vi "encodeArrayBoolean.vi"(8 "error in (no error)":errorcluster, 11 "Boolean Array":bool[](array[boolean])) -> (0 "error out":errorcluster, 3 "MessagePack":u8[](array[numeric]) format="%.0x")   [LabVIEW 2015, in "MsgPack.lvlib"]
uses:
  MsgPack.lvlib
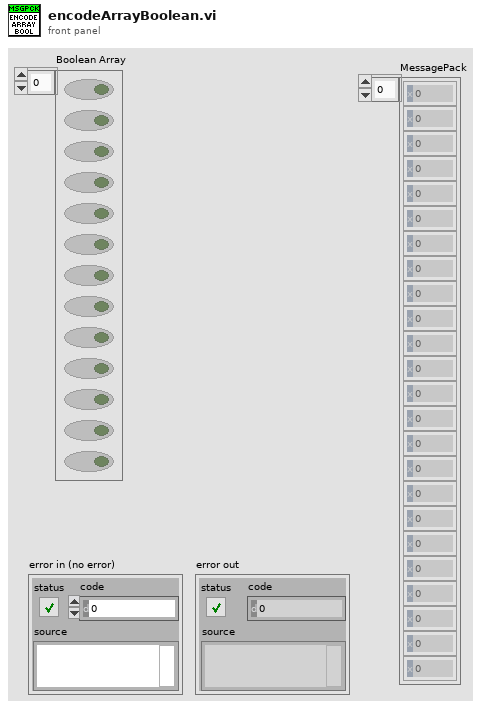
[diagram p1: front panel]
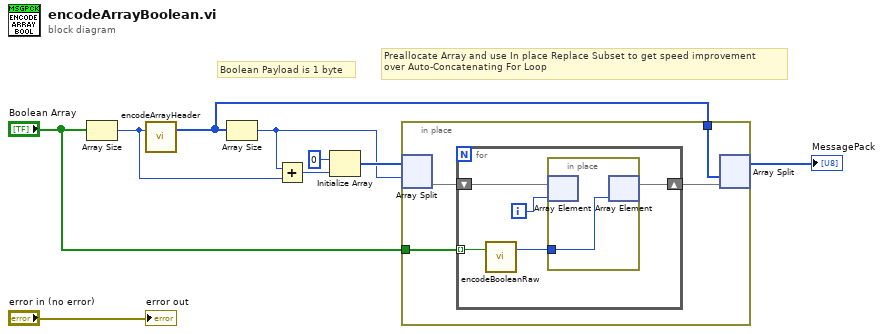
[diagram p0: block diagram]
diagram:
  # "Preallocate Array and use In place Replace Subset to get speed improvement\nover Auto-Concatenating For Loop"
  # "Boolean Payload is 1 byte"
  n1 = Array Size(array="Boolean Array") -> (size(s)=w2:i32)
  n2 = call "encodeArrayHeader.vi"("Number of Elements"=w2) -> ("array header"=w5:u8[])  [unwired: 2 in]
  n3 = Array Size(array=w5) -> (size(s)=w6:i32)
  n4 = Add(x=w6, y=w2) -> (x+y=w8:i32)
  n5 = Initialize Array(u8 0, w8) -> (w7:u8[])
  n6 = in-place {
    in-place-border: w5 -> [w13]
    in-place-border: "Boolean Array" -> [w12]
    n7 = in-place-split #1(w7, w6) -> (w11:u8[])  [unwired: 1 out]
    n8 = for {
      tunnel: w12 -> [w18] mode=indexing
      shift-right: [w14] -> w10
      shift-left: w11 -> [w16]
      i -> [w17]
      n9 = call "encodeBooleanRaw.vi"("Boolean"=w18) -> ("MessagePackRaw"=w15:u8)  [unwired: 2 in]
      n10 = in-place {
        in-place-border: w15 -> [w19]
        n11 = in-place-array #2(w16, w17) -> ()  [unwired: 1 out]
        n12 = in-place-array #2(w19) -> (w14:u8[])  [unwired: 1 out]
      }
    }
    n13 = in-place-split #1(w13, w10) -> (→"MessagePack":u8[])  [unwired: 1 out]
  }
  "error out" <- "error in (no error)"
